vi "getMagnetTarget.vi"(6 "Axis":T1=enum."Z", 8 "error in (no error)":errorcluster, 11 "Instrument.OxfordVRM in":refnum<class "Instrument.OxfordVRM.lvclass">) -> (0 "error out":errorcluster, 1 "Status":string, 2 "B Field (T)":dbl, 3 "Instrument.OxfordVRM out":refnum<class "Instrument.OxfordVRM.lvclass">, 4 "Finished?":bool)   [LabVIEW 2019, in "Instrument.OxfordVRM.lvclass"]
uses:
  Instrument.OxfordVRM.lvclass
  <userlib>/LevyLab/Instrument Framework/Instrument Types/Cryostat/Typedefs/Magnet Axis--Enum.ctl
  <userlib>/LevyLab/Instrument Framework/Instrument Types/Cryostat/Instrument.Cryostat.lvclass
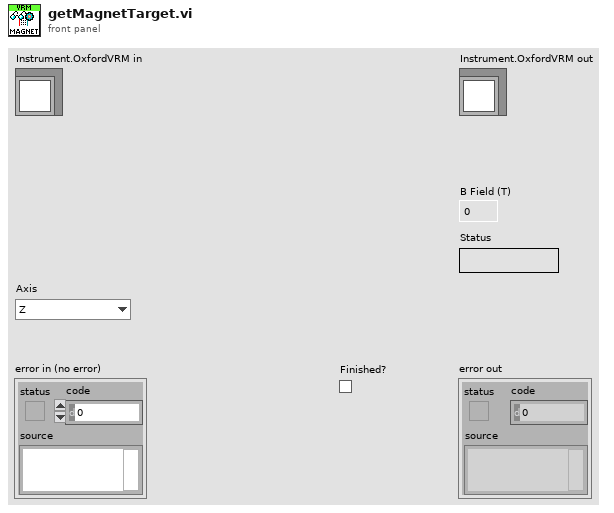
[diagram p1: front panel]
types:
  T1 = typedef "Instrument.Cryostat.lvclass/Magnet Axis--Enum.ctl" = enum16{"X", "Y", "Z"}
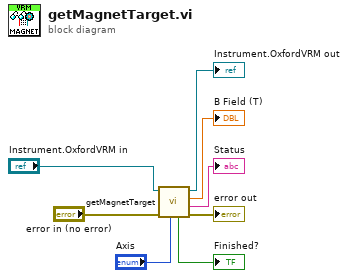
[diagram p0: block diagram]
diagram:
  n1 = call-parent "getMagnetTarget.vi"("Axis"="Axis", "error in (no error)"="error in (no error)", "Instrument.Cryostat in"="Instrument.OxfordVRM in") -> ("error out"=→"error out":errorcluster, "Status"=→"Status":string, "B Field (T)"=→"B Field (T)":dbl, "Instrument.Cryostat out"=→"Instrument.OxfordVRM out":refnum<class "Instrument.OxfordVRM.lvclass">, "Finished?"=→"Finished?":bool)  [unwired: 4 in]
